vi "assert_service_close.vi"(8 "error in (no error)":errorcluster, 11 "system.logging in":refnum<class "system.logging.lvclass">) -> (0 "error out":errorcluster)   [LabVIEW 2021, in "system.logging.lvclass"]
uses:
  system.logging.lvclass
  system.logging.lvclass/system.logging.ctl
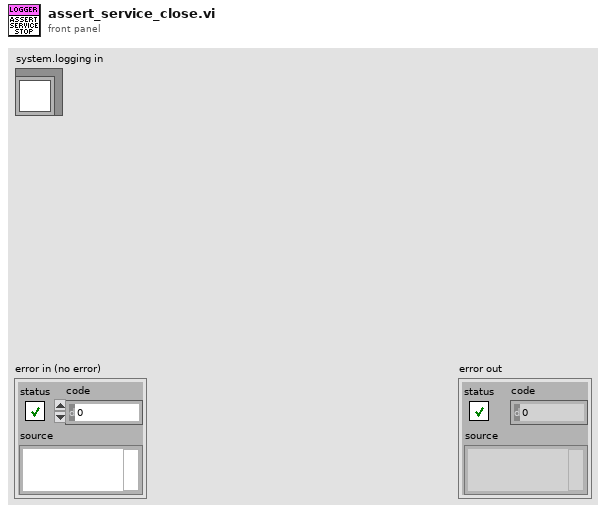
[diagram p1: front panel]
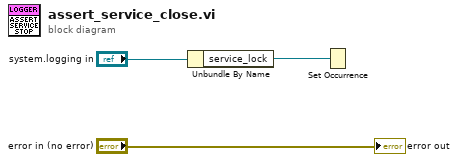
[diagram p0: block diagram]
diagram:
  n1 = Unbundle By Name("system.logging in") -> ("service_lock"=w1:refnum<k4>)
  n2 = Set Occurrence(w1) -> ()
  "error out" <- "error in (no error)"
